vi "Out_S1F18.vi"(8 "error in (no error)":errorcluster, 10 "S1F18":T1, 11 "S1 Message Class in":refnum<class "S1 Message Class.lvclass">) -> (0 "error out":errorcluster, 3 "S1 Message Class out":refnum<class "S1 Message Class.lvclass">)   [LabVIEW 2020, in "SECS Communication.lvlib" / "S1 Message Class.lvclass"]
uses:
  S1 Message Class.lvclass
  D:/Dropbox/SECS/LabVIEW Code/Com/SECS Communication/SECS-II Class/SECS-II Class.lvclass
  S1F18.ctl
  SECS-II Class/Data Message_Binary.vi
  S1 Message Class.lvclass/S1 Message Class.ctl
  SECS-II Class/SECS-II Class.lvclass
  D:/Dropbox/SECS/LabVIEW Code/Com/SECS Communication/S1 Message Class/S1 Message Class.lvclass
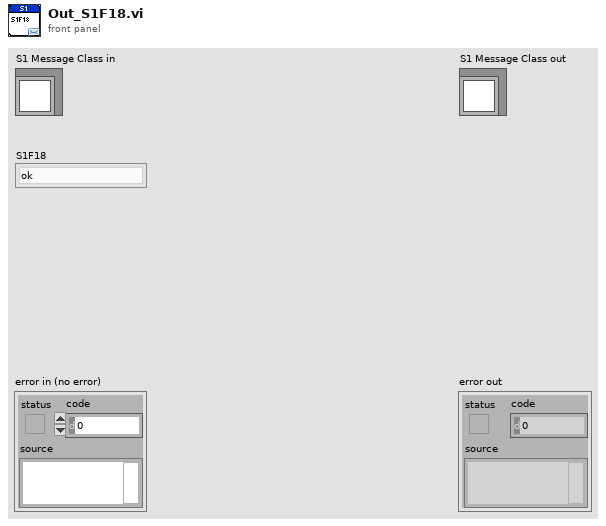
[diagram p1: front panel]
types:
  T1 = typedef "SECS Communication.lvlib/S1 Message Class.lvclass/S1F18.ctl" = enum16{"ok", "refused", "already online"}
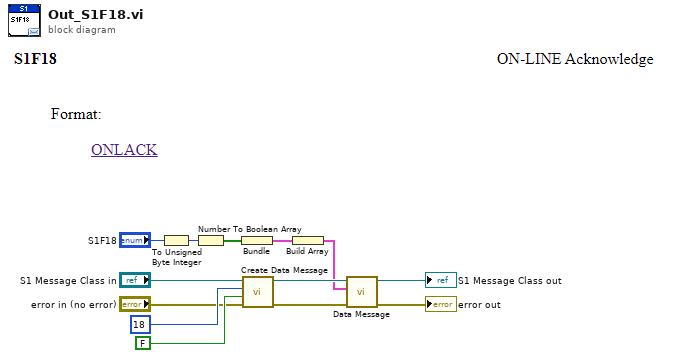
[diagram p0: block diagram]
diagram:
  n1 = To Unsigned Byte Integer(number="S1F18") -> (unsigned 8bit integer=w1:u8)
  n2 = Number To Boolean Array(number=w1) -> (Boolean array=w5:bool[])
  n3 = Bundle("Boolean array"=w5) -> (w4:cluster{"Boolean array":bool[]})  [unwired: 1 in]
  n4 = call "Create Data Message.vi"("error in (no error)"="error in (no error)", "W-Bit"=FALSE, "Function"=u8 18, "SECS-II Class in"="S1 Message Class in") -> ("error out"=w8:errorcluster, "SECS-II Class out"=w9:refnum<class "S1 Message Class.lvclass">)  [unwired: 6 in]
  n5 = Build Array(w4) -> (w3:cluster{"Boolean array":bool[]}[])
  n6 = call-poly "Data Message.vi"("error in"=w8, "Data Cluster"=w3, "SECS-II Class in"=w9) -> ("error out"=→"error out":errorcluster, "SECS-II Class out"=→"S1 Message Class out":refnum<class "S1 Message Class.lvclass">)  [unwired: 7 in]
